vi "Saturation_Indicator_Color_Code.vi"(10 "SaturationStatus":bool[](array[boolean]), 11 "IndicatorRefs":refnum<vi>[](array[refnum])) -> (3 "Error":errorcluster)   [LabVIEW 2018]
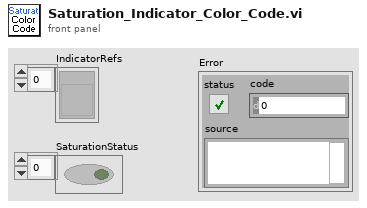
[diagram p1: front panel]
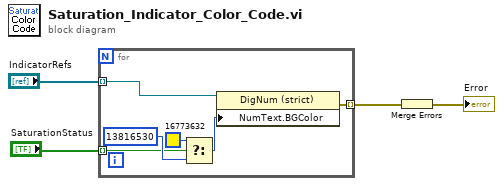
[diagram p0: block diagram]
diagram:
  n1 = for {
    tunnel: "IndicatorRefs" -> [w10] mode=indexing
    tunnel: [w9] -> w3 mode=indexing
    tunnel: "SaturationStatus" -> [w6] mode=indexing
    n2 = Select(t=u32 16773632 ("Color Box"), s=w6, f=u32 13816530 ("Label.Text Colors:BG Color")) -> (s? t:f=w5:u32)
    n3 = property on="Property Node" class="DigNum (strict)"(reference=w10, "NumText.BGColor"=w5) -> (error out=w9:errorcluster)  [unwired: 1 in, 1 out]
  }
  n4 = Merge Errors(w3) -> (→"Error":errorcluster)
